vi "Configure Channels.vi"(8 "error in (no error)":errorcluster, 11 "DI DAQmx CFG in":refnum<class "DI DAQmx Meas Freq CFG.lvclass">) -> (0 "error out":errorcluster, 3 "DI DAQmx CFG out":refnum<class "DI DAQmx Meas Freq CFG.lvclass">)   [LabVIEW 2024, in "DI DAQmx Meas Freq CFG.lvclass"]
uses:
  DI DAQmx Meas Freq CFG.lvclass
  D:/git/HAL/HAL/Configurations/CFG JSON/CFG JSON.lvclass
  D:/git/HAL/HAL/Devices/DAQmx/DAQmx Base CFG/DAQmx Base CFG.lvclass
  D:/git/HAL/HAL/Configurations/CFG Base/CFG Base.lvclass
  Configurations/CFG Base/CFG Base.lvclass/CFG Base.ctl
  DAQmx Base CFG/DAQmx Base CFG.lvclass/DAQmx Base CFG.ctl
  837b5ed5-0c17-42a6-9ee3-103f8da6f62b.vi
  <vilib>/JDP Science/JSONtext/Find Item.vi
  <vilib>/JDP Science/JSONtext/Next JSON Value.vi
  <vilib>/JDP Science/JSONtext/String Subset.vi
  <vilib>/JDP Science/JSONtext/Parsing/Advance past next JSON Value (inlined COPY).vi
  <vilib>/JDP Science/JSONtext/Parsing/Advance past whitespace.vi
  <vilib>/JDP Science/JSONtext/Parsing/Advance past String.vi
  <vilib>/JDP Science/JSONtext/Parsing/Advance past Number.vi
  <vilib>/JDP Science/JSONtext/Parsing/Advance past Line Ending.vi
  <vilib>/JDP Science/JSONtext/Parsing/Parse Full Path or Item Name.vi
  <vilib>/JDP Science/JSONtext/Parsing/Advance past Array.vi
  <vilib>/JDP Science/JSONtext/Parsing/Advance past Object.vi
  <vilib>/JDP Science/JSONtext/support/Error Cluster From Code.vi
  <vilib>/JDP Science/JSONtext/Offset/Find Item Locations by Path.vi
  <vilib>/JDP Science/JSONtext/JSON text to Variant.vi
  <vilib>/Utility/error.llb/Error Cluster From Error Code.vi
  <vilib>/DAQmx/create/channels.llb/DAQmx Create Channel (DI-Digital Input).vi
  <vilib>/JDP Science/JSONtext/LVClass Serializer/JSONtext LVClass Serializer.lvclass
  <vilib>/ErrorRing/Error Ring.xnode
  DAQmx Base CFG/DAQmx Base CFG.lvclass
  Configurations/CFG JSON/CFG JSON.lvclass
  Configurations/CFG Base/CFG Base.lvclass
panel:
  out "Line Grouping":i32(ring)=1 items=["one channel for each line", "one channel for all lines"]
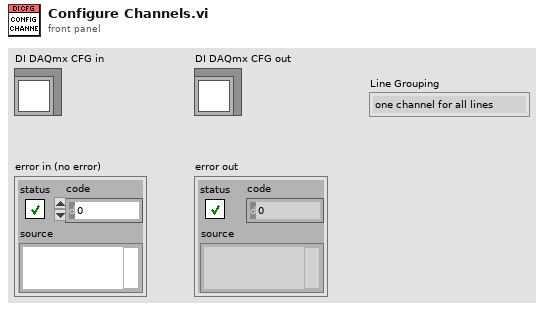
[diagram p1: front panel]
types:
  T1 = cluster{"Name":string, "Enabled":bool, "Line Grouping":string}[]
  T2 = typedef "LVStringsAndValuesArrayTypeDef_I32.ctl" = cluster{"String":string, "Value":i32}[]
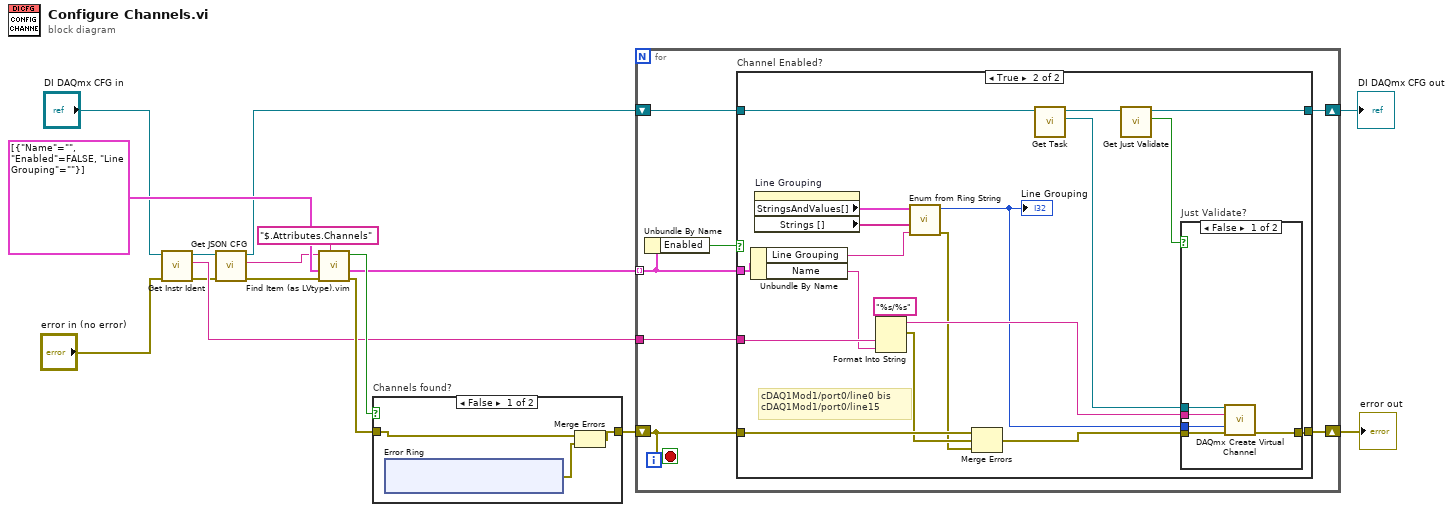
[diagram p0: block diagram]
diagram:
  n1 = call-dynamic "Get Instr Ident.vi"("error in"="error in (no error)", "CFG JSON in"="DI DAQmx CFG in") -> ("error out"=w1:errorcluster, "Instr Ident"=w7:string, "CFG JSON out"=w8:refnum<class "DI DAQmx Meas Freq CFG.lvclass">)  [unwired: 7 in]
  n2 = call "Get JSON CFG.vi"("CFG JSON in"=w8) -> ("<JSON> CFG"=w9:string, "CFG JSON out"=w6:refnum<class "DI DAQmx Meas Freq CFG.lvclass">)  [unwired: 9 in]
  n3 = call "Find Item (as LVtype).vim"("$Path or Item Name"="$.Attributes.Channels", "error in (no error)"=w1, "Data Type and Default Value"=T1 [{"Name"="", "Enabled"=FALSE, "Line Grouping"=""}], "JSON"=w9) -> ("error out"=w13:errorcluster, "Data"=w11:T1, "Found"=w14:bool)  [unwired: 4 in, 1 out]
  n4 = case "Channels found?" shown="False" w14 {
    tunnel: w13 -> [w18 w24]
    tunnel: [w16 w24] -> w12
    frame False {
      n5 = xnode "Error Ring"() -> ("error out"=w17:errorcluster)
      n6 = Merge Errors(w18, w17) -> (w16:errorcluster)
    }
    frame True {
    }
  }
  n7 = for {
    tunnel: w11 -> [w28] mode=indexing
    shift-right: [w31] -> w2
    shift-left: w12 -> [w30]
    tunnel: w7 -> [w29]
    shift-right: [w26] -> w3
    shift-left: w6 -> [w25]
    stop <- w30 stop-if-true
    n8 = Unbundle By Name(w28) -> ("Enabled"=w27:bool)
    n9 = case "Channel Enabled?" shown="True" w27 {
      tunnel: [w33 w48] -> w31
      tunnel: w30 -> [w33 w51]
      tunnel: w29 -> [_ w42]
      tunnel: w28 -> [_ w50]
      tunnel: [w32 w45] -> w26
      tunnel: w25 -> [w32 w46]
      frame False {
      }
      frame True {
        # "cDAQ1Mod1/port0/line0 bis\ncDAQ1Mod1/port0/line15"
        n10 = Unbundle By Name(w50) -> ("Line Grouping"=w36:string, "Name"=w41:string)
        n11 = property on="Line Grouping" class="Ring (strict)"() -> ("StringsAndValues[]"=w52:T2, "Strings []"=w37:string[])  [unwired: 2 in, 2 out]
        n12 = Format Into String(format string="%s/%s", w42, w41) -> (resulting string=w40:string, error out=w38:errorcluster)  [unwired: 2 in]
        n13 = call "Enum from Ring String.vi"("String to Match"=w36, "Ring Strings []"=w37, "Ring StringsAndValues[]"=w52) -> ("error out"=w34:errorcluster, "Enum Value"=w35:i32)  [unwired: 7 in]
        "Line Grouping" <- w35
        n14 = Merge Errors(w51, w38, w34) -> (w39:errorcluster)
        n15 = call "Get Task.vi"("DAQmx Base CFG in"=w46) -> ("Task"=w49:refnum<k21>, "DAQmx Base CFG out"=w47:refnum<class "DI DAQmx Meas Freq CFG.lvclass">)  [unwired: 9 in]
        n16 = call "Get Just Validate.vi"("CFG Base in"=w47) -> ("Just Validate"=w44:bool, "CFG Base out"=w45:refnum<class "DI DAQmx Meas Freq CFG.lvclass">)  [unwired: 9 in]
        n17 = case "Just Validate?" shown="False" w44 {
          tunnel: w39 -> [w57 w58]
          tunnel: w40 -> [w54 _]
          tunnel: w49 -> [w56 _]
          tunnel: [w55 w58] -> w48
          tunnel: w35 -> [w53 _]
          frame False {
            n18 = call-poly <vilib>:"DAQmx Create Virtual Channel.vi"("task in"=w56, "lines"=w54, "line grouping"=w53, "error in"=w57) -> ("error out"=w55:errorcluster)  [unwired: 10 in, 1 out]
          }
          frame True {
          }
        }
      }
    }
  }
  "error out" <- w2
  "DI DAQmx CFG out" <- w3
